vi "TP.DT.vi"(0 "Destination Address":u8, 5 "Source Address":u8=27, 7 "Sequence Number":u8=27, 9 "Data":u8[](array[numeric])) -> (4 "Arb ID":u32 format="%.0x", 8 "Data":u8[](array[numeric]))   [LabVIEW 2015, in "J1939 Addon Shared.lvlib" / "J1939 Utilities.lvlib"]
uses:
  J1939 Utilities.lvlib
  Types/PGN Fields Cluster.ctl
  Convert J1939 ID to CAN Arb ID.vi
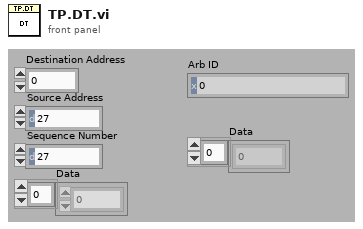
[diagram p1: front panel]
types:
  T1 = typedef "J1939 Addon Shared.lvlib/J1939 Utilities.lvlib/PGN Fields Cluster.ctl" = cluster{"Reserved Bit":u8, "Data page":u8, "PDU Format":u8, "PDU Specific":u8}
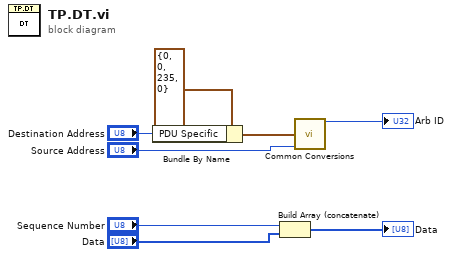
[diagram p0: block diagram]
diagram:
  n1 = Bundle By Name(cluster=T1 {"Reserved Bit"=0, "Data page"=0, "PDU Format"=235, "PDU Specific"=0} ("PGN Fields"), "PDU Specific"="Destination Address") -> (w4:T1)
  n2 = Build Array (concatenate)("Sequence Number", "Data") -> (→"Data":u8[])
  n3 = call-poly "Common Conversions.vi"("PGN Fields"=w4, "Source Address"="Source Address") -> ("ID"=→"Arb ID":u32)  [unwired: 3 in, 10 out]
